vi "Structured Light Code.vi"() -> ()   [LabVIEW 2014]
uses:
  <vilib>/vision/driver/NI_Vision_Acquisition_Software.lvlib
  <vilib>/userdefined/High Color/IMAQdx.ctl
panel:
  out "Image at Output of Vision Code":T1(plugin-control)
  out "Original Image from Camera":T1(plugin-control)
  in  "stop":bool
  out "Running Light":bool
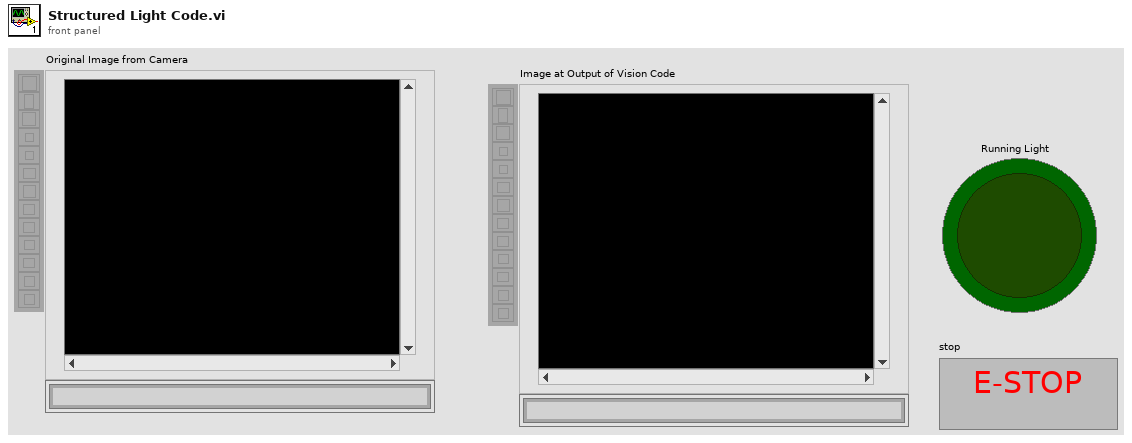
[diagram p1: front panel]
types:
  T1 = typedef "IMAQ Image.ctl" = refnum<image>
  T2 = typedef "IMAQdx.ctl" = refnum<k21>
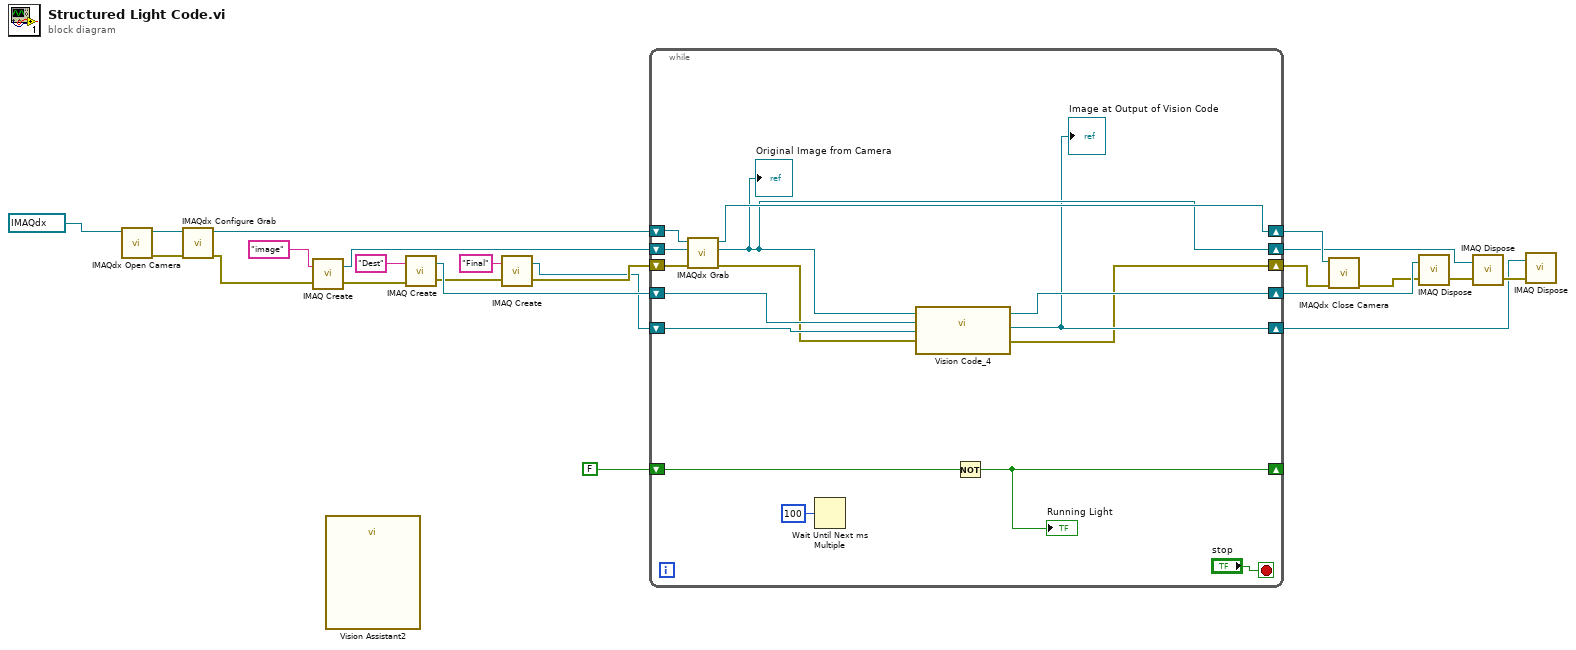
[diagram p0: block diagram]
diagram:
  n1 = call <vilib>:"IMAQdx Open Camera.vi"("Session In"=T2 "cam1") -> ("error out"=w22:errorcluster, "Session Out"=w21:T2)  [unwired: 9 in]
  n2 = call <vilib>:"IMAQdx Configure Grab.vi"("error in"=w22, "Session In"=w21) -> ("error out"=w18:errorcluster, "Session Out"=w20:T2)  [unwired: 8 in]
  n3 = call "IMAQ Create"("Image Name"="image", "error in (no error)"=w18) -> ("New Image"=w14:T1, "error out"=w16:errorcluster)  [unwired: 3 in]
  n4 = call "Vision Assistant2"() -> ()  [unwired: 24 in, 4 out]
  n5 = call "IMAQ Create"("Image Name"="Dest", "error in (no error)"=w16) -> ("New Image"=w13:T1, "error out"=w7:errorcluster)  [unwired: 3 in]
  n6 = call "IMAQ Create"("Image Name"="Final", "error in (no error)"=w7) -> ("New Image"=w4:T1, "error out"=w5:errorcluster)  [unwired: 3 in]
  n7 = while {
    shift-right: [w34] -> _
    shift-left: FALSE -> [w35]
    shift-right: [w24] -> w11
    shift-left: w5 -> [w32]
    shift-right: [w31] -> w12
    shift-left: w20 -> [w38]
    shift-right: [w30] -> w2
    shift-left: w14 -> [w37]
    shift-right: [w26] -> w10
    shift-left: w13 -> [w29]
    shift-right: [w25] -> w1
    shift-left: w4 -> [w28]
    stop <- "stop" stop-if-true
    n8 = call <vilib>:"IMAQdx Grab.vi"("error in"=w32, "Image In"=w37, "Session In"=w38) -> ("error out"=w27:errorcluster, "Image Out"=w30:T1, "Session Out"=w31:T2)  [unwired: 5 in, 1 out]
    "Original Image from Camera" <- w30
    n9 = Wait Until Next ms Multiple(millisecond multiple=u32 100) -> ()  [unwired: 1 out]
    n10 = call "Vision Code_4.vi"("Image In"=w30, "Image Dst"=w29, "Final Image Output"=w28, "error in"=w27) -> ("Image Out"=w26:T1, "Output Image"=w25:T1, "error out"=w24:errorcluster)  [unwired: 21 in]
    "Image at Output of Vision Code" <- w25
    n11 = Not(x=w35) -> (.not. x?=w34:bool)
    "Running Light" <- w34
  }
  n12 = call <vilib>:"IMAQdx Close Camera.vi"("error in"=w11, "Session In"=w12) -> ("error out"=w9:errorcluster)  [unwired: 9 in]
  n13 = call "IMAQ Dispose"("Image"=w10, "error in (no error)"=w9) -> ("error out"=w8:errorcluster)  [unwired: 4 in]
  n14 = call "IMAQ Dispose"("Image"=w2, "error in (no error)"=w8) -> ("error out"=w3:errorcluster)  [unwired: 4 in]
  n15 = call "IMAQ Dispose"("Image"=w1, "error in (no error)"=w3) -> ()  [unwired: 4 in, 1 out]
